vi "LVSgetcomportSNV.vi"() -> (0 "No Devices":bool, 1 "Port":string, 4 "Device":string)   [LabVIEW 2017]
uses:
  <vilib>/Utility/error.llb/DialogType.ctl
  instr.lib/lvserial/lvserial.lvlib
panel:
  out "Devices":string[](array[string])
  out "Ports":string[](array[string])
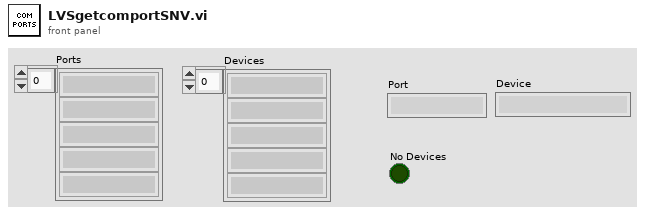
[diagram p1: front panel]
types:
  T1 = typedef "DialogType.ctl" = u16
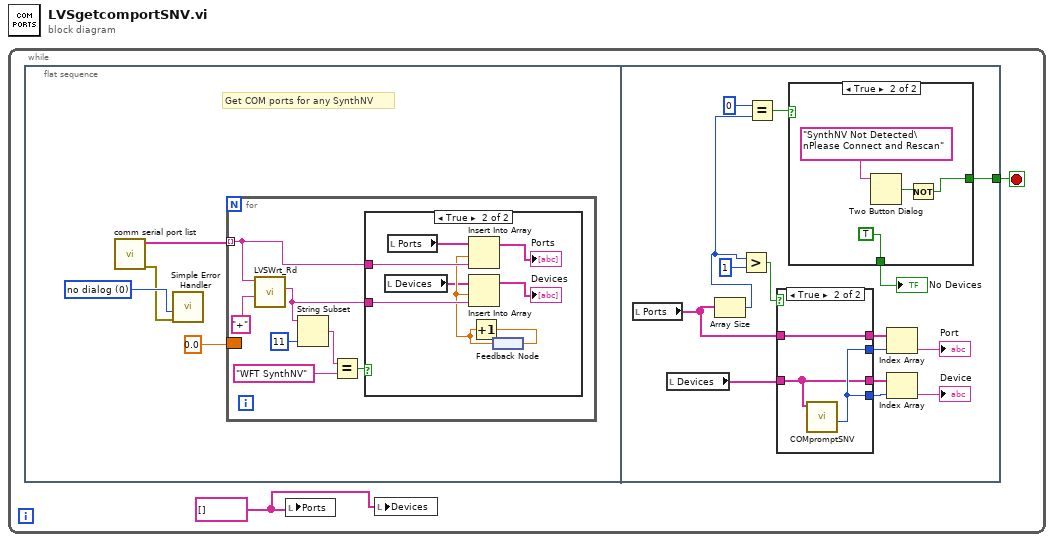
[diagram p0: block diagram]
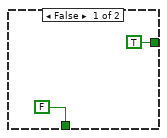
[diagram p3: hidden frame]
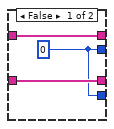
[diagram p4: hidden frame]
diagram:
  n1 = while {
    stop <- w2 stop-if-true
    w1 = string[] [] ("array")
    n2 = flat-sequence {
      tunnel: [w22] -> w2
      frame #0 {
        w6 = T1 0 items=["no dialog", "OK message", "continue or stop message", "OK message + warnings", "continue/stop + warnings"] ("type of dialog (OK msg:1)")
        # "Get COM ports for any SynthNV"
        n3 = call "comm serial port list.vi"() -> ("error out"=w3:errorcluster, "serial ports"=w4:string[])  [unwired: 10 in]
        n4 = call <vilib>:"Simple Error Handler.vi"("type of dialog (OK msg:1)"=w6, "error in (no error)"=w3) -> ()  [unwired: 8 out]
        n5 = for {
          tunnel: w4 -> [w8] mode=indexing
          border: 0.0 -> [_]
          n6 = call "LVSWrt_Rd.vi"("WriteBuf"="+" ("write buffer"), "COM Port"=w8) -> ("string read"=w7:string)  [unwired: 8 in, 1 out]
          n7 = String Subset(string=w7, length (rest)=11 ("length (rest)")) -> (substring=w11:string)  [unwired: 1 in]
          n8 = Equal?(x=w11, y="WFT SynthNV") -> (x = y?=w10:bool)
          n9 = case shown="True" w10 {
            tunnel: w7 -> [_ w21]
            tunnel: w8 -> [_ w20]
            frame False {
            }
            frame True {
              n10 = local read "Devices"() -> (w14:string[])
              n11 = local read "Ports"() -> (w15:string[])
              n12 = feedback #1() -> (w16:dbl)
              n13 = Insert Into Array(array=w15, index=w16, new element=w20) -> (→"Ports":string[])
              n14 = Insert Into Array(array=w14, index=w16, new element=w21) -> (→"Devices":string[])
              n15 = Increment(x=w16) -> (x+1=w17:dbl)
              n16 = feedback-in #1(w17) -> ()
            }
          }
        }
      }
      frame #1 {
        n17 = local read "Ports"() -> (w35:string[])
        n18 = local read "Devices"() -> (w36:string[])
        n19 = Array Size(array=w35) -> (size(s)=w32:i32)
        n20 = Greater?(x=w32, y=u32 1) -> (0:w24:bool)
        n21 = Equal?(x=0, y=w32) -> (x = y?=w31:bool)
        n22 = case shown="True" w24 {
          tunnel: w36 -> [w44 w46]
          tunnel: w35 -> [w45 w48]
          tunnel: [w45 w48] -> w26
          tunnel: [w43 w47] -> w27
          tunnel: [w44 w46] -> w28
          tunnel: [w43 w47] -> w29
          frame False {
            w43 = 0 ("Numeric")
          }
          frame True {
            n23 = call "COMpromptSNV.vi"("Devices"=w46) -> ("Numeric"=w47:i32)  [unwired: 10 in]
          }
        }
        n24 = case shown="True" w31 {
          tunnel: [FALSE TRUE] -> w34
          tunnel: [TRUE w39] -> w22
          frame False {
          }
          frame True {
            n25 = Two Button Dialog(message="SynthNV Not Detected\nPlease Connect and Rescan") -> (T button?=w42:bool)  [unwired: 2 in]
            n26 = Not(x=w42) -> (.not. x?=w39:bool)
          }
        }
        "No Devices" <- w34
        n27 = Index Array(array=w26, index=w27) -> (element=→"Port":string)
        n28 = Index Array(array=w28, index=w29) -> (element=→"Device":string)
      }
    }
    n29 = local write "Ports"(w1) -> ()
    n30 = local write "Devices"(w1) -> ()
  }
